vi "Set VI Relative Position.vi"(11 "Wire in":refnum<vi>) -> (3 "Relative Position":T1)   [LabVIEW 2017]
uses:
  <vilib>/_script/New VI Object TypeDefs/NewVIObject_LVRelativePositionTypeDef.ctl
  <vilib>/_script/New VI Object TypeDefs/NewVIObject_LVRelativeDirectionTypeDef.ctl
  <vilib>/Utility/miscctls.llb/LVPoint32TypeDef.ctl
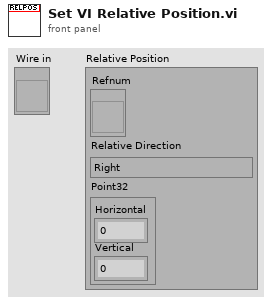
[diagram p1: front panel]
types:
  T1 = typedef "NewVIObject_LVRelativePositionTypeDef.ctl" = cluster{"Refnum":refnum<vi>, "Relative Direction":T2, "Point32":T3}
  T2 = typedef "NewVIObject_LVRelativeDirectionTypeDef.ctl" = enum32{"Right", "Left", "Top", "Bottom", "Top Right", "Top Left", "Bottom Right", "Bottom Left"}
  T3 = typedef "LVPoint32TypeDef.ctl" = cluster{"Horizontal":i32, "Vertical":i32}
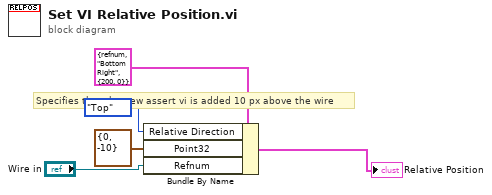
[diagram p0: block diagram]
diagram:
  # "Specifies that the new assert vi is added 10 px above the wire"
  n1 = Bundle By Name(cluster=T1 {"Refnum"=refnum, "Relative Direction"=enum."Bottom Right", "Point32"={"Horizontal"=200, "Vertical"=0}} ("Relative Position"), "Relative Direction"=NewVIObject_LVRelativeDirectionTypeDef."Top", "Point32"=T3 {"Horizontal"=0, "Vertical"=-10}, "Refnum"="Wire in") -> (→"Relative Position":T1)
